vi "OP500_NEW CSV READER_P.vi"(6 "errin":errorcluster, 8 "DCIR+ ?":bool, 9 "Choisir le fichier CSV":path) -> (0 "sortie d'erreur":errorcluster, 3 "cluster":T1)   [LabVIEW 2020]
uses:
  <vilib>/Utility/file.llb/Read Delimited Spreadsheet (DBL).vi
panel:
  out "DCIR+ mOhm":dbl
  out "all rows":dbl[][](array[numeric]) caption="toutes les lignes"
  out "DTC":dbl
  out "SOH":dbl
  out "SOC":dbl
  out "NTC Min":dbl
  out "NTC Max":dbl
  out "VCell Min":dbl
  out "VCell Max":dbl
  out "Average Current":dbl
  out "sous-tableau":dbl[](array[numeric])
  out "DCIR- mOhm":dbl
  out "OCV Pack":dbl
  out "Tension fin DCIR":dbl
  out "Chaîne":string
  out "Temps de la décharge (seconde)":i32
  # "This VI can analyse the CSV file generated by labview only, not lithium balance file"
  # "1"
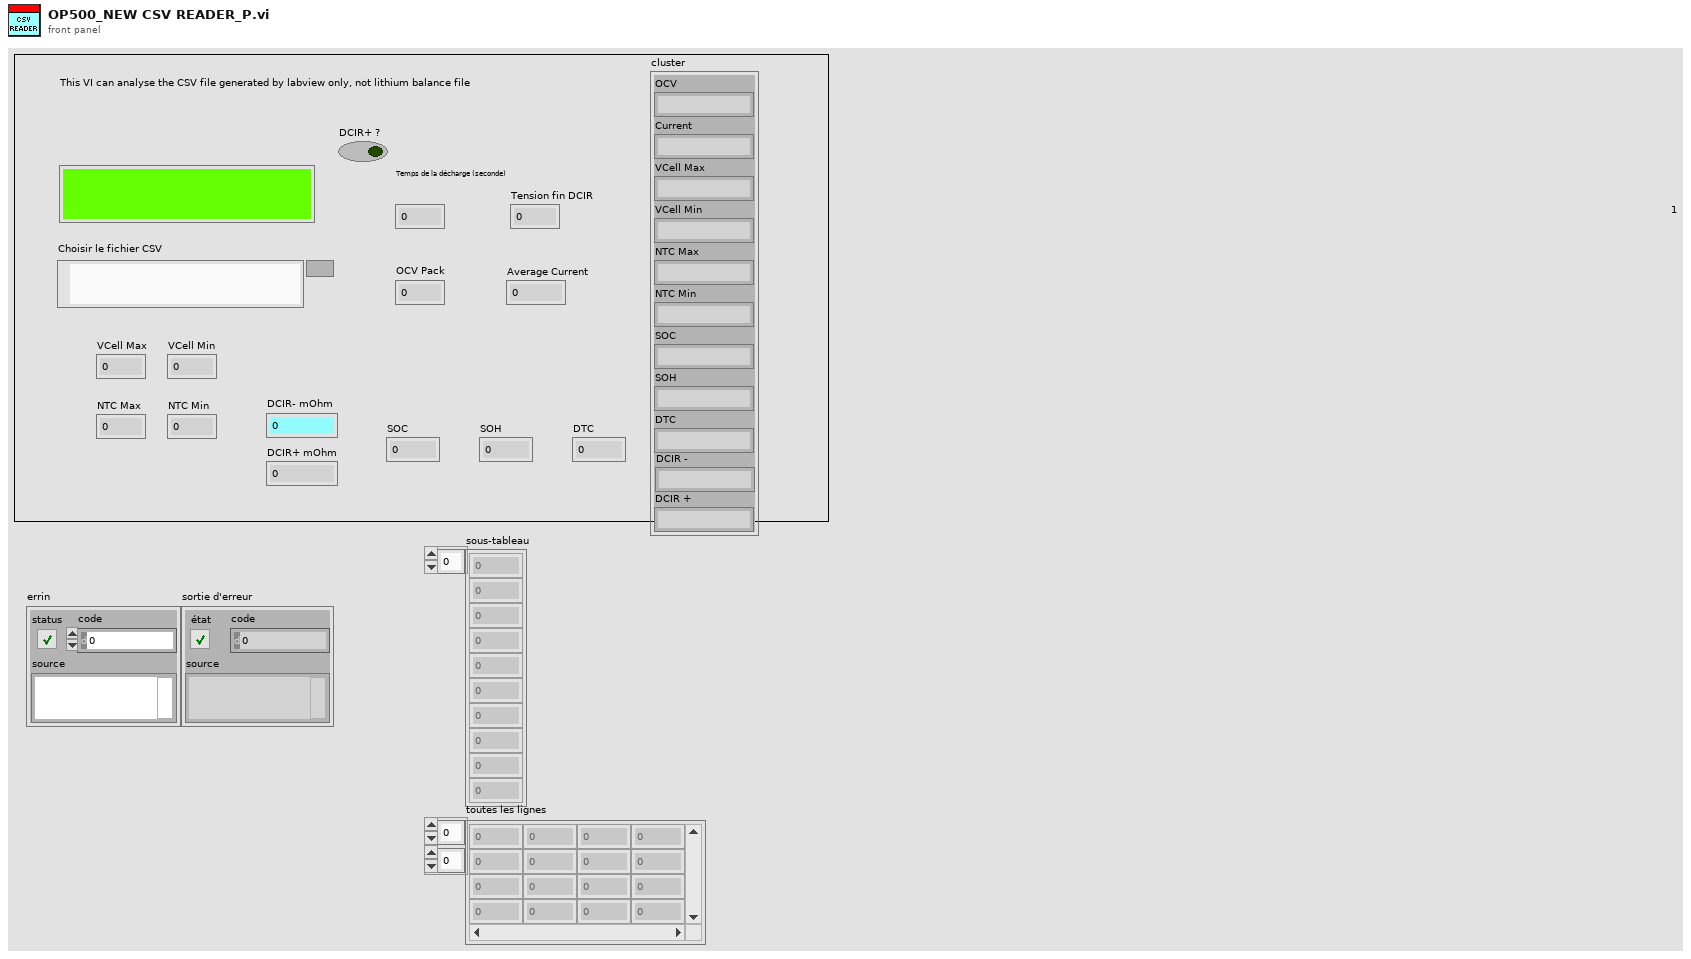
[diagram p1: front panel]
types:
  T1 = cluster{"OCV":string, "Current":string, "VCell Max":string, "VCell Min":string, "NTC Max":string, "NTC Min":string, "SOC":string, "SOH":string, "DTC":string, "DCIR -":string, "DCIR +":string}
  T2 = cluster{"[0]":string, "[1]":string, "[2]":string, "[3]":string, "[4]":string, "[5]":string, "[6]":string, "[7]":string, "[8]":string, "[9]":string, "[10]":string}
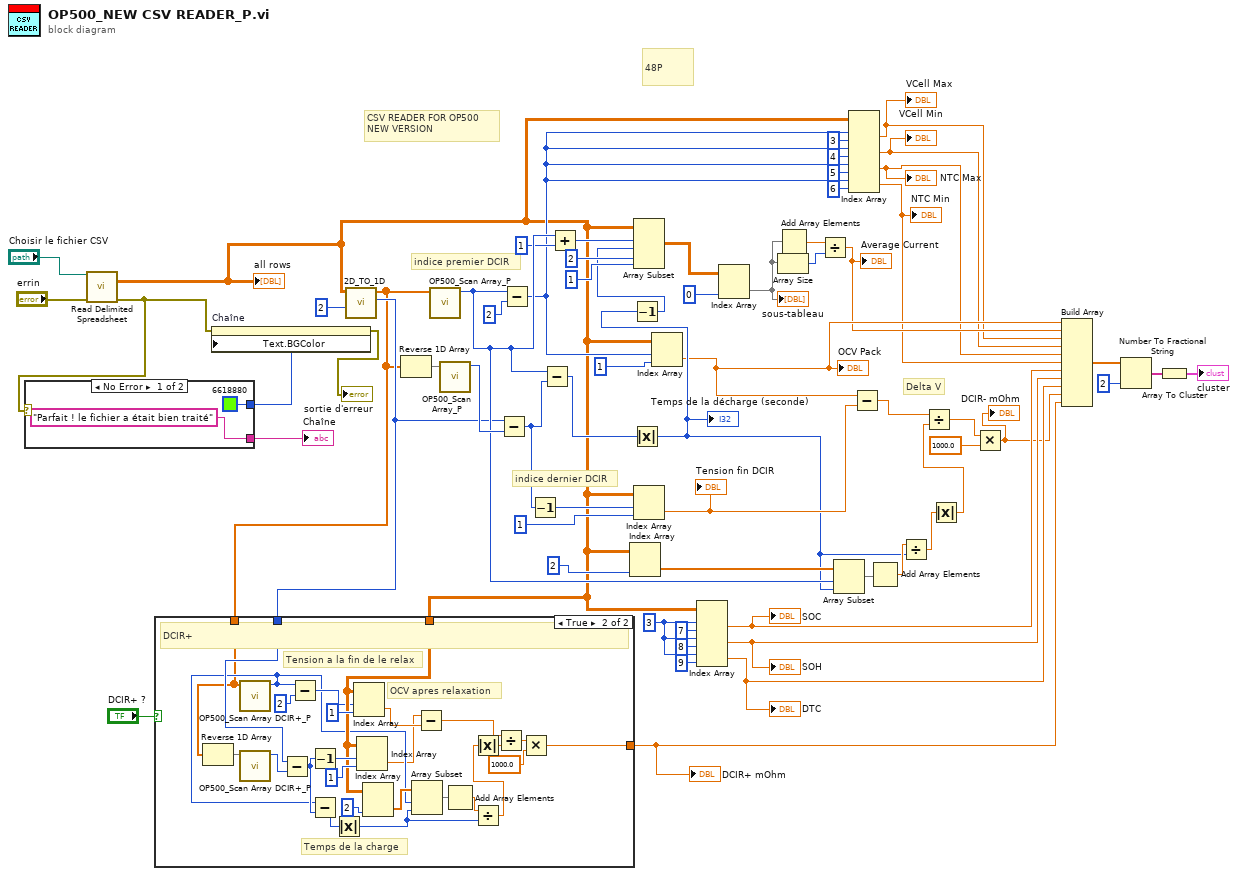
[diagram p0: block diagram]
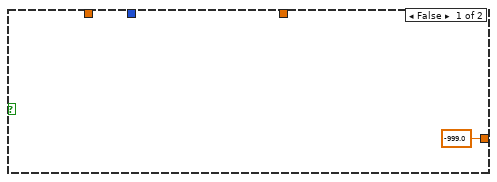
[diagram p2: hidden frame]
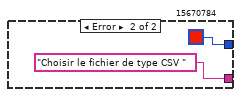
[diagram p3: hidden frame]
diagram:
  w19 = 3 ("indice (ligne)")
  # "48P"
  # "indice dernier DCIR"
  # "indice premier DCIR"
  # "CSV READER FOR OP500 \nNEW VERSION"
  # "Delta V"
  n1 = call-poly <vilib>:"Read Delimited Spreadsheet.vi"("file path (dialog if empty)"="Choisir le fichier CSV", "error in (no error)"="errin") -> ("all rows"=w5:dbl[][], "error out"=w7:errorcluster)  [unwired: 8 in, 4 out]
  "all rows" <- w5
  n2 = case shown="No Error" w7 {
    tunnel: ["Parfait ! le fichier a était bien traité" ("Chaîne") "Choisir le fichier de type CSV " ("Chaîne")] -> w62
    tunnel: [u32 6618880 ("Texte.Couleurs du texte:Arrière-plan") u32 15670784 ("Texte.Couleurs du texte:Arrière-plan")] -> w61
    frame No Error {
    }
    frame Error {
    }
  }
  "Chaîne" <- w62
  n3 = property on="Chaîne" class="Str"(error in=w7, "Text.BGColor"=w61) -> (error out=→"sortie d'erreur":errorcluster)  [unwired: 1 in, 1 out]
  n4 = call "2D_TO_1D.vi"("indice colonne courant"=2, "Array 2D"=w5) -> ("Array1D size"=w4:i32, "Array 1D"=w1:dbl[])  [unwired: 8 in]
  n5 = case shown="True" "DCIR+ ?" {
    tunnel: w1 -> [_ w71]
    tunnel: w5 -> [_ w90]
    tunnel: w4 -> [_ w94]
    tunnel: [-999.0 w74] -> w3
    frame False {
    }
    frame True {
      # "OCV apres relaxation"
      # "Temps de la charge"
      # "Tension a la fin de le relax"
      # "DCIR+"
      n6 = Reverse 1D Array(array=w71) -> (reversed array=w72:dbl[])
      n7 = call "OP500_Scan Array DCIR+_P.vi"("Array"=w71) -> ("Indice du premier valeur du courant DCIR"=w79:i32)  [unwired: 10 in]
      n8 = call "OP500_Scan Array DCIR+_P.vi"("Array"=w72) -> ("Indice du premier valeur du courant DCIR"=w73:i32)  [unwired: 10 in]
      n9 = Subtract(x=w94, y=w73) -> (x-y=w91:i32)
      n10 = Subtract(x=w79, y=2) -> (x-y=w87:i32)
      n11 = Decrement(x=w91) -> (x-1=w93:i32)
      n12 = Subtract(x=w79, y=w91) -> (x-y=w78:i32)
      n13 = Absolute Value(x=w78) -> (abs(x)=w77:i32)
      n14 = Index Array(array=w90, index (row)=w87, index (col)=1 ("disabled index (col)")) -> (element=w76:dbl)
      n15 = Index Array(array=w90, index (row)=w93, index (col)=1 ("disabled index (col)")) -> (element=w75:dbl)
      n16 = Index Array(array=w90, index (col)=2 ("disabled index (col)")) -> (element=w88:dbl[])  [unwired: 1 in]
      n17 = Array Subset(array=w88, index=w79, length=w77) -> (w86:dbl[])
      n18 = Subtract(x=w75, y=w76) -> (x-y=w82:dbl)
      n19 = Add Array Elements(numeric array=w86) -> (sum=w85:dbl)
      n20 = Divide(x=w85, y=w77) -> (x/y=w84:dbl)
      n21 = Absolute Value(x=w84) -> (abs(x)=w83:dbl)
      n22 = Divide(x=w82, y=w83) -> (x/y=w81:dbl)
      n23 = Multiply(x=w81, y=1000.0) -> (x*y=w74:dbl)
    }
  }
  "DCIR+ mOhm" <- w3
  n24 = Reverse 1D Array(array=w1) -> (reversed array=w2:dbl[])
  n25 = call "OP500_Scan Array_P.vi"("Array"=w1) -> ("Indice du premier valeur du courant DCIR"=w43:i32)  [unwired: 10 in]
  n26 = call "OP500_Scan Array_P.vi"("Array"=w2) -> ("Indice du premier valeur du courant DCIR"=w46:i32)  [unwired: 10 in]
  n27 = Subtract(x=w4, y=w46) -> (x-y=w64:i32)
  n28 = Subtract(x=w43, y=2) -> (x-y=w30:i32)
  n29 = Decrement(x=w64) -> (x-1=w60:i32)
  n30 = Subtract(x=w43, y=w64) -> (x-y=w63:i32)
  n31 = Add(x=w43, y=1) -> (x+y=w44:i32)
  n32 = Index Array(array=w5, index (col)=2 ("indice désactivé (col)")) -> (element=w56:dbl[])  [unwired: 1 in]
  n33 = Absolute Value(x=w63) -> (abs(x)=w39:i32)
  "Temps de la décharge (seconde)" <- w39
  n34 = Decrement(x=w39) -> (x-1=w38:i32)
  n35 = Array Subset(array=w5, index (row)=w44, length (row)=w38, index (col)=2 ("indice"), length (col)=1 ("longueur")) -> (w37:dbl[][])
  n36 = Index Array(array=w5, index (row)=w60, index (col)=1 ("length")) -> (element=w58:dbl)
  "Tension fin DCIR" <- w58
  n37 = Index Array(array=w5, index (row)=w30, index (col)=1 ("indice")) -> (element=w27:dbl)
  "OCV Pack" <- w27
  n38 = Index Array(array=w5, index (row) #1=w19, index (col) #1=7 ("indice désactivé (col)"), index (row) #2=w19, index (col) #2=8 ("indice désactivé (col)"), index (row) #3=w19, index (col) #3=9 ("indice désactivé (col)")) -> (element #1=w17:dbl, element #2=w16:dbl, element #3=w15:dbl)
  "SOC" <- w17
  "SOH" <- w16
  "DTC" <- w15
  n39 = Index Array(array=w37, index (col)=0 ("indice désactivé (col)")) -> (element=w35:dbl[])  [unwired: 1 in]
  "sous-tableau" <- w35
  n40 = Array Size(array=w35) -> (size(s)=w33:i32)
  n41 = Add Array Elements(numeric array=w35) -> (sum=w34:dbl)
  n42 = Divide(x=w34, y=w33) -> (x/y=w26:dbl)
  "Average Current" <- w26
  n43 = Array Subset(array=w56, index=w43, length=w39) -> (w55:dbl[])
  n44 = Index Array(array=w5, index (row) #1=w30, index (col) #1=3 ("indice désactivé (col)"), index (row) #2=w30, index (col) #2=4 ("indice désactivé (col)"), index (row) #3=w30, index (col) #3=5 ("indice désactivé (col)"), index (row) #4=w30, index (col) #4=6 ("indice désactivé (col)")) -> (element #1=w25:dbl, element #2=w24:dbl, element #3=w23:dbl, element #4=w22:dbl)
  "VCell Max" <- w25
  "VCell Min" <- w24
  "NTC Max" <- w23
  "NTC Min" <- w22
  n45 = Subtract(x=w27, y=w58) -> (x-y=w54:dbl)
  n46 = Add Array Elements(numeric array=w55) -> (sum=w49:dbl)
  n47 = Divide(x=w49, y=w39) -> (x/y=w51:dbl)
  n48 = Absolute Value(x=w51) -> (abs(x)=w50:dbl)
  n49 = Divide(x=w54, y=w50) -> (x/y=w53:dbl)
  n50 = Multiply(x=w53, y=1000.0) -> (x*y=w10:dbl)
  "DCIR- mOhm" <- w10
  n51 = Build Array(w27, w26, w25, w24, w23, w22, w17, w16, w15, w10, w3) -> (w14:dbl[])
  n52 = Number To Fractional String(number=w14, precision (6)=i16 2 ("précision (6)")) -> (F-format string=w12:string[])  [unwired: 2 in]
  n53 = Array To Cluster(array=w12) -> (cluster=→"cluster":T2)
